vi "MARS_MagnetometerHMC588L_I2C_Open.vi"(8 "error in":errorcluster, 10 "I2C Bus":T3, 11 "Controller":T4) -> (0 "error out":errorcluster, 3 "I2CDevRef":T1={"DevStatus"={"status"=FALSE, "code"=0, "source"=""}, "Controller"=enum."Controller 1", "Device Address"=0, "Handle"=0, "I2C Bus"=enum."Invalid"} {"Device Address" format="%.0x"})   [LabVIEW 2014]
uses:
  <vilib>/Rock Robotics/SystemInterfaces/Typedef/FPGA_TypedefAnalogModule.ctl
  <vilib>/Rock Robotics/SystemInterfaces/i2clib/i2c_bus.ctl
  <vilib>/Rock Robotics/WPI/I2C/WPI_I2CDevRef.ctl
  <vilib>/Rock Robotics/SystemInterfaces/Typedef/FPGA_TypedefDigitalModule.ctl
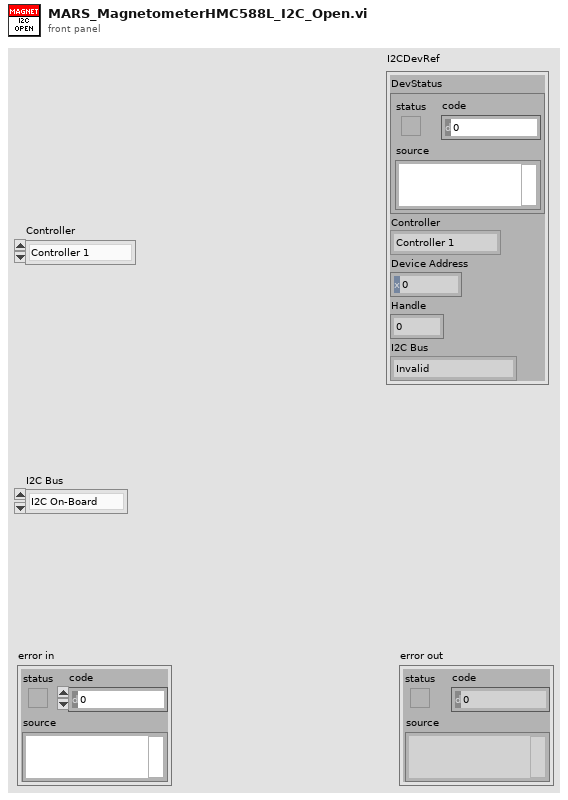
[diagram p1: front panel]
types:
  T1 = typedef "WPI_I2CDevRef.ctl" = cluster{"DevStatus":errorcluster, "Controller":T2, "Device Address":u8, "Handle":i32, "I2C Bus":T3}
  T2 = typedef "FPGA_TypedefDigitalModule.ctl" = enum16{"Controller 1"}
  T3 = typedef "i2c_bus.ctl" = enum16{"I2C On-Board", "I2C MXP", "Invalid"}
  T4 = typedef "FPGA_TypedefAnalogModule.ctl" = enum16{"Controller 1"}
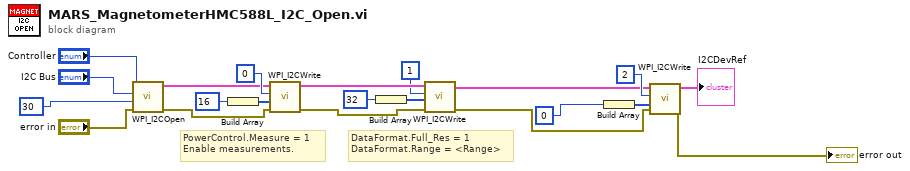
[diagram p0: block diagram]
diagram:
  # "DataFormat.Full_Res = 1\nDataFormat.Range = <Range>"
  # "PowerControl.Measure = 1\nEnable measurements."
  n1 = call <vilib>:"WPI_I2COpen.vi"("error in"="error in", "Device Address"=u8 30 ("Data To Send"), "I2C Bus"="I2C Bus", "Controller"="Controller") -> ("error out"=w3:errorcluster, "I2CDevRef"=w16:T1)  [unwired: 6 out]
  n2 = Build Array(u8 16 ("Data To Send")) -> (w19:u8[])
  n3 = call <vilib>:"WPI_I2CWrite.vi"("error in (no error)"=w3, "I2CDataToSend"=w19, "I2CRegister"=u8 0 ("Data To Send"), "I2CDevRef"=w16) -> ("error out"=w2:errorcluster, "I2CDevRef"=w8:T1)  [unwired: 6 out]
  n4 = Build Array(u8 32 ("Data To Send")) -> (w5:u8[])
  n5 = call <vilib>:"WPI_I2CWrite.vi"("error in (no error)"=w2, "I2CDataToSend"=w5, "I2CRegister"=u8 1 ("Data To Send"), "I2CDevRef"=w8) -> ("error out"=w1:errorcluster, "I2CDevRef"=w9:T1)  [unwired: 6 out]
  n6 = Build Array(u8 0 ("Data To Send")) -> (w20:u8[])
  n7 = call <vilib>:"WPI_I2CWrite.vi"("error in (no error)"=w1, "I2CDataToSend"=w20, "I2CRegister"=u8 2 ("Data To Send"), "I2CDevRef"=w9) -> ("error out"=→"error out":errorcluster, "I2CDevRef"=→"I2CDevRef":T1)  [unwired: 6 out]
